vi "Read Key STR.vi"(7 "Section Name":string, 8 "error in":errorcluster, 9 "default value":string, 10 "Key Name":string, 11 "Config Cluster in":T1) -> (0 "error out":errorcluster, 1 "Value":string, 2 "Found?":bool, 3 "Config Cluster out":T1)   [LabVIEW 2017]
uses:
  Config Cluster.ctl
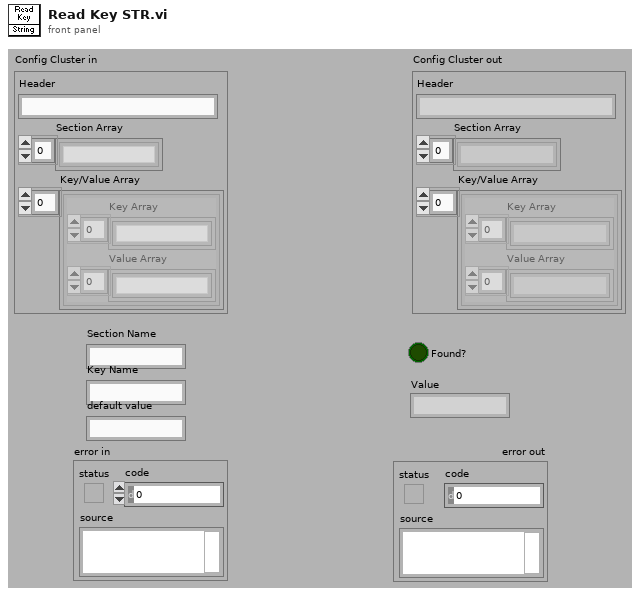
[diagram p1: front panel]
types:
  T1 = typedef "Config Cluster.ctl" = cluster{"Header":string, "Section Array":string[], "Key/Value Array":cluster{"Key Array":string[], "Value Array":string[]}[]}
  T2 = cluster{"Key Array":string[], "Value Array":string[]}[]
  T3 = cluster{"Key Array":string[], "Value Array":string[]}
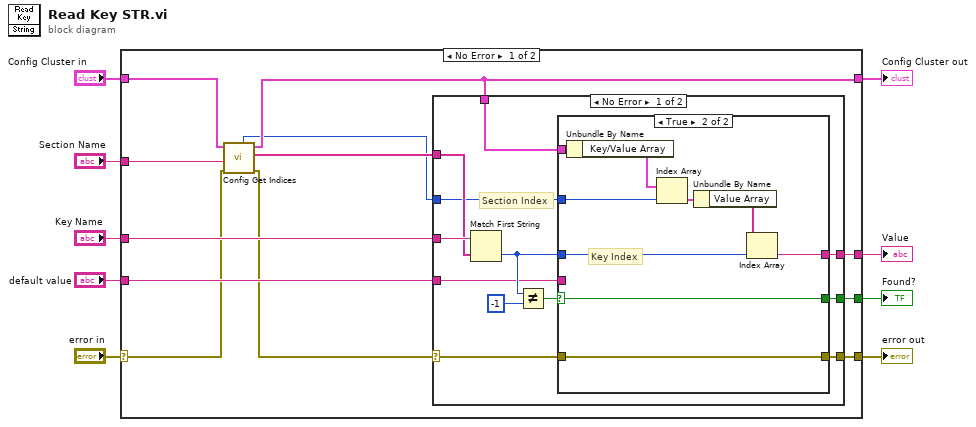
[diagram p0: block diagram]
diagram:
  n1 = case shown="No Error" "error in" {
    selector: "error in" -> [w16 w49]
    tunnel: [w13 w49] -> w8
    tunnel: "Config Cluster in" -> [w14 w50]
    tunnel: [w12 w50] -> w6
    tunnel: "Section Name" -> [w18 _]
    tunnel: "Key Name" -> [w21 _]
    tunnel: [w20 w48] -> w3
    tunnel: "default value" -> [w19 w48]
    tunnel: [w10 _] -> w1
    frame No Error {
      n2 = call "Config Get Indices.vi"("error in"=w16, "Section Name"=w18, "Config Cluster in"=w14) -> ("error out"=w17:errorcluster, "Key Array"=w15:string[], "Config Cluster out"=w12:T1, "Section Index"=w11:i32)  [unwired: 4 in, 1 out]
      n3 = case shown="No Error" w17 {
        selector: w17 -> [w29 w46]
        tunnel: w21 -> [w33 _]
        tunnel: [w24 w47] -> w20
        tunnel: w19 -> [w23 w47]
        tunnel: w15 -> [w31 _]
        tunnel: [w28 w46] -> w13
        tunnel: w12 -> [w26 _]
        tunnel: w11 -> [w25 _]
        tunnel: [w22 _] -> w10
        frame No Error {
          # "Section Index"
          n4 = Match First String(2:w31, 3:w33) -> (0:w27:i32)  [unwired: 1 out]
          n5 = Not Equal?(x=w27, y=-1) -> (x != y?=w30:bool)
          n6 = case shown="True" w30 {
            selector: w30 -> [w34 w37]
            tunnel: w29 -> [w35 w38]
            tunnel: [w35 w38] -> w28
            tunnel: w27 -> [_ w40]
            tunnel: w26 -> [_ w45]
            tunnel: w25 -> [_ w43]
            tunnel: [w36 w39] -> w24
            tunnel: w23 -> [w36 _]
            tunnel: [w34 w37] -> w22
            frame False {
            }
            frame True {
              # "Key Index"
              n7 = Unbundle By Name(w45) -> ("Key/Value Array"=w44:T2)
              n8 = Index Array(array=w44, index=w43) -> (element=w42:T3)
              n9 = Unbundle By Name(w42) -> ("Value Array"=w41:string[])
              n10 = Index Array(array=w41, index=w40) -> (element=w39:string)
            }
          }
        }
        frame Error {
        }
      }
    }
    frame Error {
    }
  }
  "error out" <- w8
  "Config Cluster out" <- w6
  "Value" <- w3
  "Found?" <- w1
